vi "butterworth filter (SubVI).vi"(1 "Array 2":dbl[][](array[numeric]), 2 "w":dbl) -> (0 "Array":dbl[][](array[numeric]))   [LabVIEW 2009]
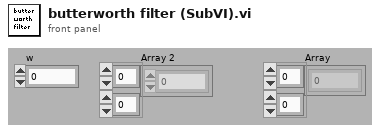
[diagram p1: front panel]
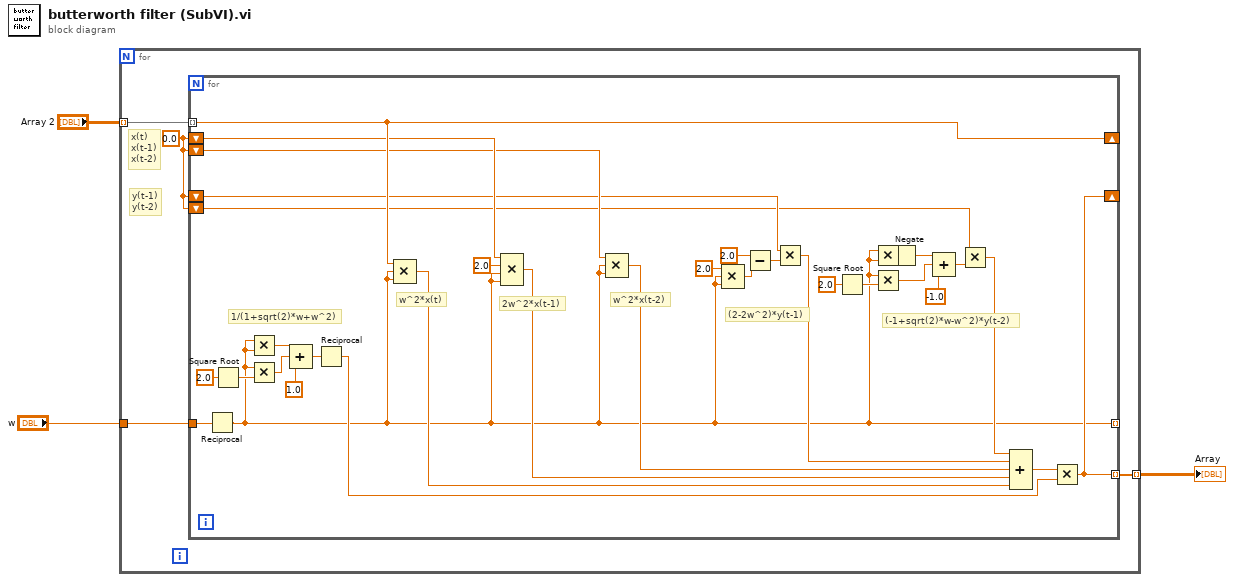
[diagram p0: block diagram]
diagram:
  n1 = for {
    tunnel: "Array 2" -> [w7] mode=indexing
    tunnel: [w5] -> w3 mode=indexing
    tunnel: "w" -> [w4]
    w6 = 0.0
    # "y(t-1)\ny(t-2)"
    # "x(t)\nx(t-1)\nx(t-2)"
    n2 = for {
      tunnel: w7 -> [w36] mode=indexing
      shift-right: [w36] -> _
      shift-left: w6 -> [w13]
      shift-left: w6 -> [w12]
      shift-right: [w14] -> _
      shift-left: w6 -> [w11]
      shift-left: w6 -> [w10]
      tunnel: [w8] -> _ mode=indexing
      tunnel: [w14] -> w5 mode=indexing
      tunnel: w4 -> [w9]
      # "(2-2w^2)*y(t-1)"
      # "(-1+sqrt(2)*w-w^2)*y(t-2)"
      # "w^2*x(t-2)"
      # "2w^2*x(t-1)"
      # "w^2*x(t)"
      # "1/(1+sqrt(2)*w+w^2)"
      n3 = Reciprocal(x=w9) -> (1/x=w8:dbl)
      n4 = Square Root(x=2.0 ("y")) -> (sqrt(x)=w33:dbl)
      n5 = Multiply(x=w8, y=w8) -> (x*y=w40:dbl)
      n6 = Multiply(x=w8, y=w33) -> (x*y=w39:dbl)
      n7 = Compound Arithmetic op=unknown(w40, w39, 1.0 ("y")) -> (w37:dbl)
      n8 = Reciprocal(x=w37) -> (1/x=w15:dbl)
      n9 = Compound Arithmetic op=MULTIPLY(w36, w8, w8) -> (w17:dbl)
      n10 = Compound Arithmetic op=MULTIPLY(w13, 2.0 ("y"), w8, w8) -> (w18:dbl)
      n11 = Compound Arithmetic op=MULTIPLY(w12, w8, w8) -> (w19:dbl)
      n12 = Compound Arithmetic op=MULTIPLY(2.0 ("value"), w8, w8) -> (w24:dbl)
      n13 = Subtract(x=2.0 ("value"), y=w24) -> (x-y=w22:dbl)
      n14 = Multiply(x=w11, y=w22) -> (x*y=w20:dbl)
      n15 = Square Root(x=2.0 ("y")) -> (sqrt(x)=w32:dbl)
      n16 = Multiply(x=w8, y=w8) -> (x*y=w29:dbl)
      n17 = Multiply(x=w8, y=w32) -> (x*y=w30:dbl)
      n18 = Negate(x=w29) -> (-x=w27:dbl)
      n19 = Compound Arithmetic op=unknown(w27, w30, -1.0 ("y")) -> (w26:dbl)
      n20 = Multiply(x=w10, y=w26) -> (x*y=w21:dbl)
      n21 = Compound Arithmetic op=ADD(w21, w20, w19, w18, w17) -> (w16:dbl)
      n22 = Multiply(x=w16, y=w15) -> (x*y=w14:dbl)
    }
  }
  "Array" <- w3
